vi "Drive Controller.vi"(8 "error in":errorcluster) -> ()   [LabVIEW 2015]
doc: "This VI executes continuously carrying out the current operation and responding to updates or new operation requests. It will often contain the timing or control code that is difficult to place directly in TeleOp. This VI generally opens all sensors and motors and isolates the rest of the robot code from knowing implementation details of how the operations are carried out."
uses:
  Drive Setpoints.ctl
  Drive Operations.ctl
  <vilib>/Rock Robotics/WPI/SafetyOutput/WPI_SafetyOutputConfigMenu.ctl
  <vilib>/Rock Robotics/SystemInterfaces/DIO/FPGA_DIOPWMChannel.ctl
  <vilib>/Rock Robotics/WPI/RobotDrive/WPI_RobotDriveOpen4MotorWithTalon.vi
panel:
  out "Setpoints":T1(graph)
  out "Current\nCmd":string
  # "Tip: It may be helpful to observe inputs and sensor values.\nYou may also want to display tuning or debugging controls."
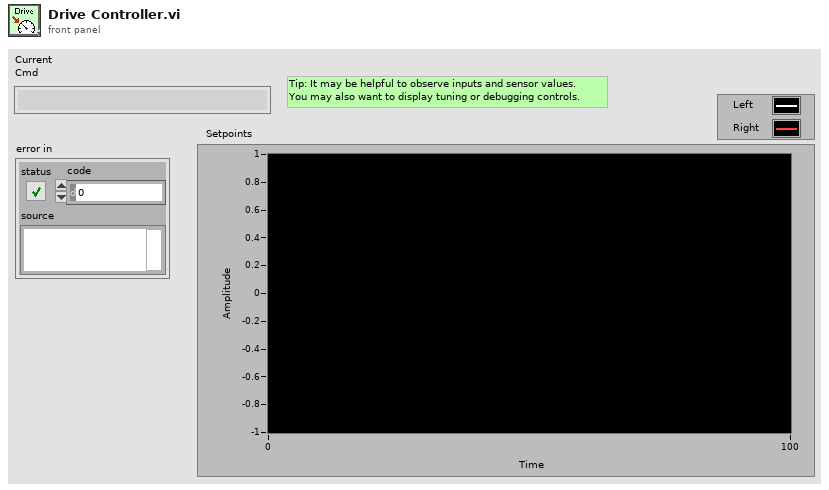
[diagram p1: front panel]
types:
  T1 = cluster{"Left Setpoint":dbl, "Right Setpoint":dbl}
  T2 = typedef "FPGA_DIOPWMChannel.ctl" = enum8{"PWM 0", "PWM 1", "PWM 2", "PWM 3", "PWM 4", "PWM 5", "PWM 6", "PWM 7", "PWM 8", "PWM 9", "PWM MXP 0", "PWM MXP 1", "PWM MXP 2", "PWM MXP 3", "PWM MXP 4", "PWM MXP 5", "PWM MXP 6", "PWM MXP 7", "PWM MXP 8", "PWM MXP 9", "Invalid"}
  T3 = typedef "WPI_SafetyOutputConfigMenu.ctl" = enum16{"Enable", "Disable"}
  T4 = typedef "Drive Setpoints.ctl" = cluster{"Operation":T5, "Left Setpoint":dbl, "Right Setpoint":dbl, "Duration":dbl}
  T5 = typedef "Drive Operations.ctl" = enum16{"Reserve", "Read Current", "Immediate", "Drive for Time", "Drive for Distance"}
  T6 = typedef "WPI_RobotDriveDevRef.ctl" = cluster{"DevStatus":errorcluster, "Motors[]":T7[], "Square Inputs":bool, "Max Output":dbl}
  T7 = typedef "WPI_MotorControlDeviceRef.ctl" = cluster{"DeviceStatus":errorcluster, "Type":T8, "PWM":cluster{"PWM Channel":T2, "DeadBand":T9}, "CAN":cluster{"Device Number":u8, "Control Mode":T10, "Semaphore":T11, "Max Vout":dbl, "TalonSRX Control Mode":T12}, "Invert":bool}
  T8 = typedef "WPI_MotorControlType.ctl" = enum16{"PWM", "CAN", "CANTalonSRX"}
  T9 = typedef "WPI_PWMDeadband.ctl" = cluster{"Name":string, "maxPositivePwm":i32, "minPositivePwm":i32, "centerPwm":i32, "maxNegativePwm":i32, "minNegativePwm":i32, "angularRange":u16}
  T10 = typedef "WPI_CANJaguar_ControlMode.ctl" = enum8{"Percent VBus", "Current", "Speed", "Position", "Voltage"}
  T11 = typedef "Semaphore RefNum" = refnum<k1>
  T12 = typedef "WPI_CANTalonSRX_APIControlMode.ctl" = enum8{"Percent VBus", "Speed", "Position", "Slave", "Unchanged / Invalid", "Voltage Compensation", "Current", "Motion Profile"}
  T13 = typedef "Command Status Info.ctl" = cluster{"Name":string, "Status":T14, "notifier out":T15}
  T14 = typedef "Completion Status.ctl" = enum16{"Successful", "Aborted", "Incomplete"}
  T15 = typedef "Completion Notifier.ctl" = refnum<notifier>
  T16 = cluster{"SubSystem Data":T4, cluster{"Start Time (ms)":u32, "Iterations":i32}, cluster{"Command Info":T13, "Description":string, "SubSystem Data":T4, "notifier out":refnum<notifier>, "Subsystem Name":string}}
  T17 = cluster{"SubSystem Data":T4, cluster{"Start Time (ms)":u32, "Iterations":i32}, "Default Command Arguments":cluster{"Command Info":T13, "Description":string, "SubSystem Data":T4, "notifier out":refnum<notifier>, "Subsystem Name":string}}
  T18 = cluster{"Don't move motors while reserved":dbl, "Don't move motors while reserved":dbl}
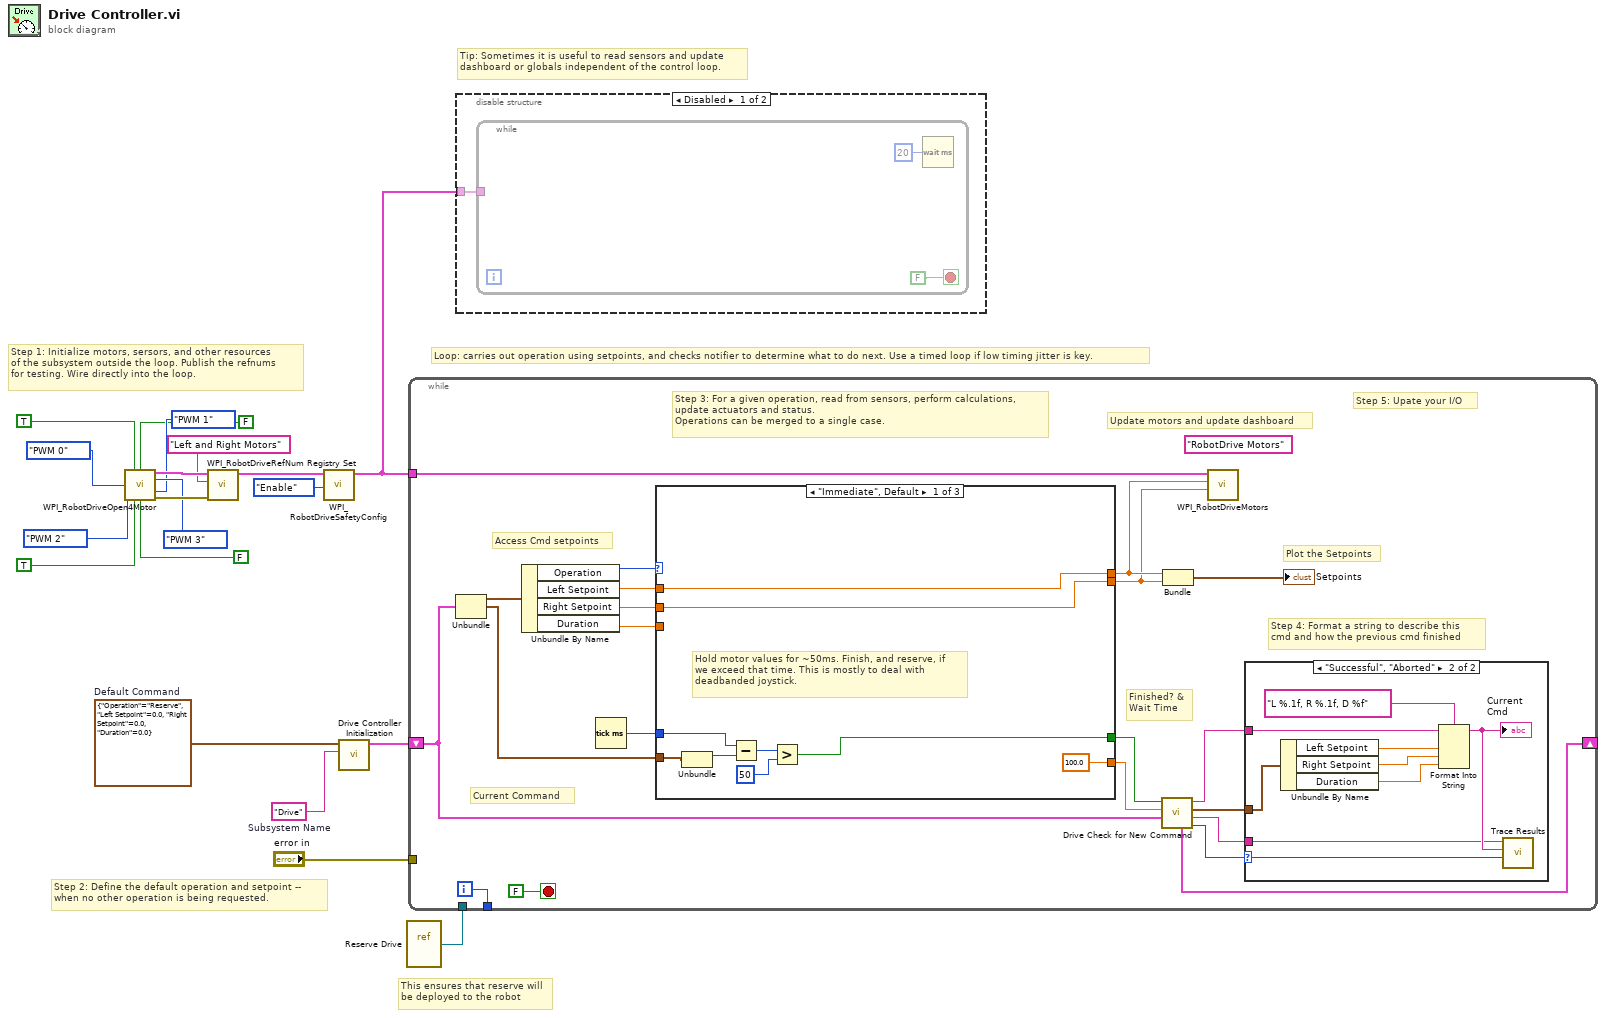
[diagram p0: block diagram]
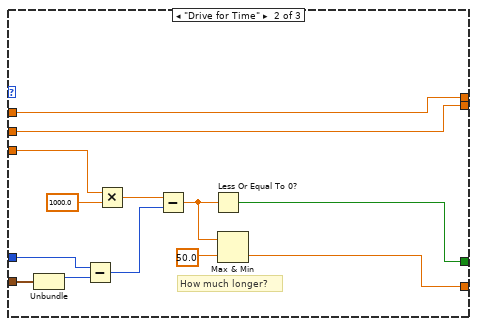
[diagram p4: hidden frame]
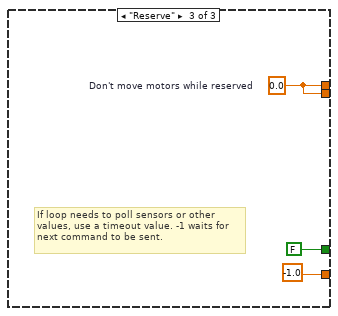
[diagram p5: hidden frame]
diagram:
  w18 = T4 {"Operation"=enum."Reserve", "Left Setpoint"=0.0, "Right Setpoint"=0.0, "Duration"=0.0}  # Default Command
  w19 = "Drive"  # Subsystem Name
  # "This ensures that reserve will\nbe deployed to the robot"
  # "Tip: Sometimes it is useful to read sensors and update\ndashboard or globals independent of the control loop."
  # "Step 2: Define the default operation and setpoint --\nwhen no other operation is being requested."
  # "Step 1: Initialize motors, sersors, and other resources\nof the subsystem outside the loop. Publish the refnums\nfor testing. Wire directly into the loop."
  # "Loop: carries out operation using setpoints, and checks notifier to determine what to do next. Use a timed loop if low timing jitter is key."
  n1 = call-poly <vilib>:"WPI_RobotDriveOpen4Motor.vi"("Rear Left Motor"=FPGA_DIOPWMChannel."PWM 2", "Rear Left Motor Inverted"=TRUE, "Rear Right Motor Inverted"=FALSE, "Rear Right Motor"=FPGA_DIOPWMChannel."PWM 3", "Front Left Motor"=FPGA_DIOPWMChannel."PWM 0", "Front Right Motor"=FPGA_DIOPWMChannel."PWM 1", "Front Left Motor Inverted"=TRUE, "Front Right Motor Inverted"=FALSE) -> ("RobotDriveDevRef"=w17:T6, "error out"=w15:errorcluster)  [unwired: 6 in]
  n2 = call <vilib>:"WPI_RobotDriveRefNum Registry Set.vi"("error in (no error)"=w15, "refnum name"="Left and Right Motors", "RobotDriveDevRef"=w17) -> ("RobotDriveDevRef"=w14:T6)  [unwired: 1 in, 7 out]
  n3 = call <vilib>:"WPI_RobotDriveSafetyConfig.vi"("mode"=WPI_SafetyOutputConfigMenu."Enable", "RobotDriveDevRef"=w14) -> ("RobotDriveDevRef"=w12:T6)  [unwired: 8 in, 1 out]
  n4 = call "Drive Controller Initialization.vi"("Subsystem Name"=w19, "Default Command"=w18) -> ("output cluster"=w10:T16)  [unwired: 9 in]
  n5 = vi-ref "Reserve Drive.vi"() -> (w9:refnum<vi>)
  n6 = while {
    shift-right: [w27] -> _
    shift-left: w10 -> [w20]
    tunnel: [w39] -> _
    tunnel: w12 -> [w35]
    tunnel: "error in" -> [_]
    tunnel: w9 -> [_]
    i -> [w39]
    stop <- FALSE stop-if-true
    (unwired) "RobotDrive Motors" ("Name")
    # "Step 5: Upate your I/O"
    # "Step 4: Format a string to describe this\ncmd and how the previous cmd finished"
    # "Current Command"
    # "Update motors and update dashboard"
    # "Plot the Setpoints"
    # "Access Cmd setpoints"
    # "Finished? &\nWait Time"
    # "Step 3: For a given operation, read from sensors, perform calculations,\nupdate actuators and status.\nOperations can be merged to a single case."
    n7 = Unbundle(w20) -> ("SubSystem Data"=w34:T4, w21:cluster{"Start Time (ms)":u32, "Iterations":i32})  [unwired: 1 out]
    n8 = Unbundle By Name(w34) -> ("Operation"=w33:T5, "Left Setpoint"=w32:dbl, "Right Setpoint"=w31:dbl, "Duration"=w30:dbl)
    n9 = Tick Count (ms)() -> (millisecond timer value=w29:u32)
    n10 = case shown="\"Immediate\", Default" w33 {
      tunnel: [100.0 w59 -1.0] -> w26
      tunnel: [w51 w66 FALSE ("ignore previous (F)")] -> w25
      tunnel: w21 -> [w50 w68 _]
      tunnel: [w57 w65 w72] -> w37
      tunnel: [w56 w64 w72] -> w36
      tunnel: w32 -> [w57 w65 _]
      tunnel: w31 -> [w56 w64 _]
      tunnel: w30 -> [_ w63 _]
      tunnel: w29 -> [w52 w62 _]
      frame "Immediate", Default {
        # "Hold motor values for ~50ms. Finish, and reserve, if\nwe exceed that time. This is mostly to deal with\ndeadbanded joystick."
        n11 = Unbundle(w50) -> ("Start Time (ms)"=w53:u32)  [unwired: 1 out]
        n12 = Subtract(x=w52, y=w53) -> (x-y=w54:u32)
        n13 = Greater?(x=w54, y=u8 50 ("Left Motor")) -> (0:w51:bool)
      }
      frame "Drive for Time" {
        # "How much longer?"
        n14 = Unbundle(w68) -> ("Start Time (ms)"=w67:u32)  [unwired: 1 out]
        n15 = Subtract(x=w62, y=w67) -> (x-y=w71:u32)
        n16 = Multiply(x=w63, y=1000.0) -> (x*y=w70:dbl)
        n17 = Subtract(x=w70, y=w71) -> (x-y=w61:dbl)
        n18 = Less Or Equal To 0?(x=w61) -> (x <= 0?=w66:bool)
        n19 = Max & Min(x=w61, y=50.0) -> (min(x,y)=w59:dbl)  [unwired: 1 out]
      }
      frame "Reserve" {
        w72 = 0.0  # Don't move motors while reserved
        # "If loop needs to poll sensors or other\nvalues, use a timeout value. -1 waits for\nnext command to be sent."
      }
    }
    n20 = call "Drive Check for New Command.vi"("input cluster"=w20, "Wait time (ms)"=w26, "Finished?"=w25) -> ("Completion"=w28:T14, "Subsystem Name"=w22:string, "SetPoint"=w23:T4, "Initial Trace String"=w24:string, "output cluster"=w27:T17)  [unwired: 4 in]
    n21 = Bundle("Don't move motors while reserved"=w37, "Don't move motors while reserved"=w36) -> (→"Setpoints":T18)  [unwired: 1 in]
    n22 = call <vilib>:"WPI_RobotDriveMotors.vi"("RightSpeed"=w36, "LeftSpeed"=w37, "RobotDriveDevRef"=w35) -> ()  [unwired: 1 in, 8 out]
    n23 = case shown="\"Successful\", \"Aborted\"" w28 {
      selector: w28 -> [_ w49]
      tunnel: w24 -> [_ w44]
      tunnel: w23 -> [_ w45]
      tunnel: w22 -> [_ w41]
      frame "Incomplete", Default {
        # "Continuing current command"
      }
      frame "Successful", "Aborted" {
        # "Report and setup for next command"
        n24 = Unbundle By Name(w45) -> ("Left Setpoint"=w47:dbl, "Right Setpoint"=w48:dbl, "Duration"=w42:dbl)
        n25 = Format Into String(format string="L %.1f, R %.1f, D %f", initial string=w44, w47, w48, w42) -> (resulting string=w43:string)  [unwired: 1 in, 1 out]
        "Current\nCmd" <- w43
        n26 = call <vilib>:"Trace Results.vi"("Status of previous command"=w49, "Description"=w43, "Subsystem"=w41) -> ()  [unwired: 9 in]
      }
    }
  }
  n27 = disable-structure shown="Disabled" {
    disable-tunnel: w12 -> [w75 _]
    frame Disabled {
      n28 = while {
        tunnel: w75 -> [_]
        stop <- FALSE stop-if-true
        n29 = Wait (ms)(milliseconds to wait=u32 20) -> ()  [unwired: 1 out]
      }
    }
    frame Enabled {
    }
  }
